vi "Profile Auton - Drive distance with encoders.vi"(8 "error in (no error)":errorcluster) -> (0 "error out":errorcluster)   [LabVIEW 2017]
uses:
  Auton Control.ctl
  <vilib>/Rock Robotics/WPI/ThirdParty/Phoenix-LabVIEW/Motor Controller/Get/CTRE_Phoenix_MotorController_GetSelectedSensorData.vi
panel:
  in  "Cluster":T1 {"Shooting Mode" items=["No Shooter", "Low Shooter", "High Shooter"]}
  out "Right":dbl
  out "Left":dbl
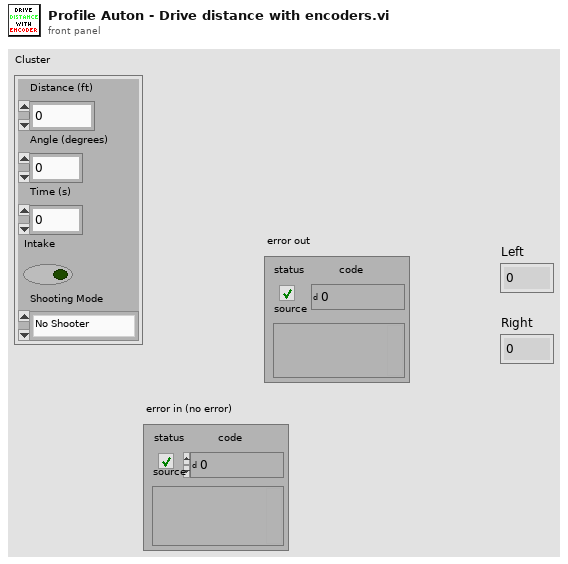
[diagram p1: front panel]
types:
  T1 = typedef "Auton Control.ctl" = cluster{"Distance (ft)":dbl, "Angle (degrees)":dbl, "Time (s)":dbl, "Intake":bool, "Shooting Mode":u16}
  T2 = typedef "WPI_MotorControlDeviceRef.ctl" = cluster{"DeviceStatus":errorcluster, "Type":T3, "PWM":cluster{"PWM Channel":T4, "DeadBand":T5}, "CAN":cluster{"Device Number":u8, "SetOutput VI Ref":variant, "GetOutput VI Ref":variant, "Enable VI Ref":variant, "Disable VI Ref":variant, "Data":variant}, "Invert":bool, "DIO PWM":cluster{"PWM \"Enable\" Channel":T4, "DIOChannel":T6, "PWM Rate":dbl}}
  T3 = typedef "WPI_MotorControlType.ctl" = enum16{"PWM", "CAN", "DIO PWM"}
  T4 = typedef "FPGA_DIOPWMChannel.ctl" = enum8{"PWM 0", "PWM 1", "PWM 2", "PWM 3", "PWM 4", "PWM 5", "PWM 6", "PWM 7", "PWM 8", "PWM 9", "PWM MXP 0", "PWM MXP 1", "PWM MXP 2", "PWM MXP 3", "PWM MXP 4", "PWM MXP 5", "PWM MXP 6", "PWM MXP 7", "PWM MXP 8", "PWM MXP 9", "Invalid"}
  T5 = typedef "WPI_PWMDeadband.ctl" = cluster{"Name":string, "maxPositivePwm":i32, "minPositivePwm":i32, "centerPwm":i32, "maxNegativePwm":i32, "minNegativePwm":i32, "angularRange":u16}
  T6 = typedef "FPGA_DIOChannel.ctl" = enum8{"DIO 0", "DIO 1", "DIO 2", "DIO 3", "DIO 4", "DIO 5", "DIO 6", "DIO 7", "DIO 8", "DIO 9", "DIO MXP 0", "DIO MXP 1", "DIO MXP 2", "DIO MXP 3", "DIO MXP 4", "DIO MXP 5", "DIO MXP 6", "DIO MXP 7", "DIO MXP 8", "DIO MXP 9", "DIO MXP 10", "DIO MXP 11", "DIO MXP 12", "DIO MXP 13", "DIO MXP 14", "DIO MXP 15", "SPI Port CS1", "SPI Port CS2", "SPI Port CS3", "SPI Port MISO", "SPI Port MOSI", "Invalid"}
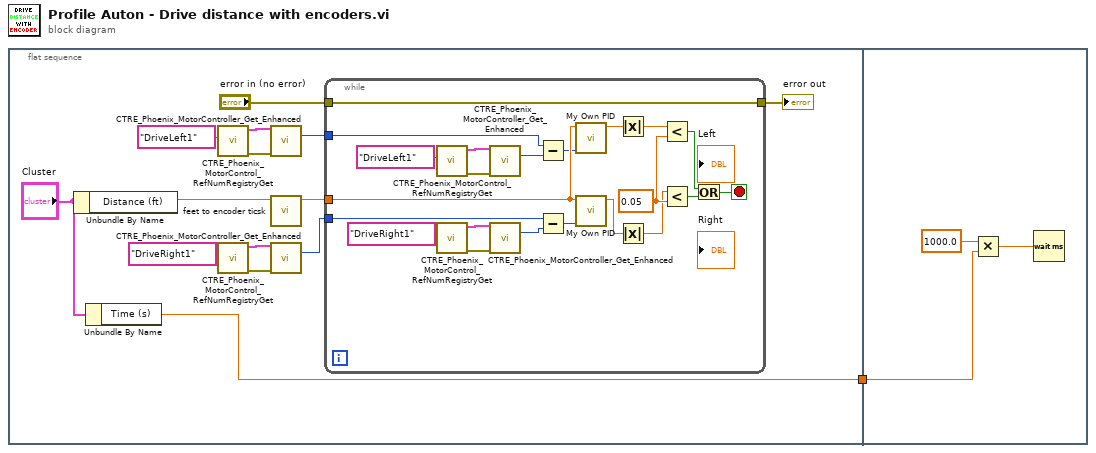
[diagram p0: block diagram]
diagram:
  n1 = flat-sequence {
    tunnel: [w2] -> w1
    tunnel: w1 -> [w39]
    frame #0 {
      n2 = Unbundle By Name("Cluster") -> ("Distance (ft)"=w4:dbl)
      n3 = Unbundle By Name("Cluster") -> ("Time (s)"=w2:dbl)
      n4 = call <vilib>:"CTRE_Phoenix_MotorControl_RefNumRegistryGet.vi"("refnum name"="DriveLeft1") -> ("error out"=w10:errorcluster, "PhoenixMotorControlDevRef"=w14:T2)  [unwired: 9 in]
      n5 = call <vilib>:"CTRE_Phoenix_MotorControl_RefNumRegistryGet.vi"("refnum name"="DriveRight1") -> ("error out"=w9:errorcluster, "PhoenixMotorControlDevRef"=w11:T2)  [unwired: 9 in]
      n6 = call-poly <vilib>:"CTRE_Phoenix_MotorController_Get_Enhanced.vi"("PhoenixMotorControlDevRef"=w14, "error in"=w10) -> ("Position (Raw Sensor Units)"=w8:i32)  [unwired: 10 in, 3 out]
      n7 = call "feet to encoder ticsk.vi"("Distance in feet wanted"=w4) -> ("Encoder Ticks"=w15:dbl)  [unwired: 10 in]
      n8 = call-poly <vilib>:"CTRE_Phoenix_MotorController_Get_Enhanced.vi"("PhoenixMotorControlDevRef"=w11, "error in"=w9) -> ("Position (Raw Sensor Units)"=w7:i32)  [unwired: 10 in, 3 out]
      n9 = while {
        tunnel: w15 -> [w37]
        tunnel: w8 -> [w30]
        tunnel: w7 -> [w28]
        tunnel: [w20] -> w6
        tunnel: "error in (no error)" -> [w20]
        stop <- w24 stop-if-true
        w23 = 0.05
        n10 = call <vilib>:"CTRE_Phoenix_MotorControl_RefNumRegistryGet.vi"("refnum name"="DriveLeft1") -> ("error out"=w35:errorcluster, "PhoenixMotorControlDevRef"=w31:T2)  [unwired: 9 in]
        n11 = call <vilib>:"CTRE_Phoenix_MotorControl_RefNumRegistryGet.vi"("refnum name"="DriveRight1") -> ("error out"=w36:errorcluster, "PhoenixMotorControlDevRef"=w34:T2)  [unwired: 9 in]
        n12 = call-poly <vilib>:"CTRE_Phoenix_MotorController_Get_Enhanced.vi"("PhoenixMotorControlDevRef"=w31, "error in"=w35) -> ("Position (Raw Sensor Units)"=w29:i32)  [unwired: 10 in, 3 out]
        n13 = call-poly <vilib>:"CTRE_Phoenix_MotorController_Get_Enhanced.vi"("PhoenixMotorControlDevRef"=w34, "error in"=w36) -> ("Position (Raw Sensor Units)"=w27:i32)  [unwired: 10 in, 3 out]
        n14 = Subtract(x=w30, y=w29) -> (x-y=w26:i32)
        n15 = Subtract(x=w28, y=w27) -> (x-y=w25:i32)
        n16 = call "My Own PID.vi"("Current Input"=w26, "Wanted End"=w37) -> ("Output"=w17:dbl)  [unwired: 9 in]
        n17 = call "My Own PID.vi"("Current Input"=w25, "Wanted End"=w37) -> ("Output"=w19:dbl)  [unwired: 9 in]
        n18 = Absolute Value(x=w17) -> (abs(x)=w16:dbl)
        n19 = Absolute Value(x=w19) -> (abs(x)=w18:dbl)
        n20 = Less?(x=w16, y=w23) -> (x < y?=w22:bool)
        n21 = Less?(x=w18, y=w23) -> (x < y?=w21:bool)
        n22 = Or(x=w22, y=w21) -> (x .or. y?=w24:bool)
      }
      "error out" <- w6
    }
    frame #1 {
      n23 = Multiply(x=1000.0, y=w39) -> (x*y=w40:dbl)
      n24 = Wait (ms)(milliseconds to wait=w40) -> ()  [unwired: 1 out]
    }
  }
